vi "局部小信号变比.vi"(4 "长度":i32, 5 "数据":u8[](array[numeric]) format="%.0x") -> (3 "小信号变比":cluster{"UB":sgl, "IB":sgl, "UC":sgl, "IA":sgl})   [LabVIEW 2014]
panel:
  out "数组":u8[](array[numeric]) format="%x"
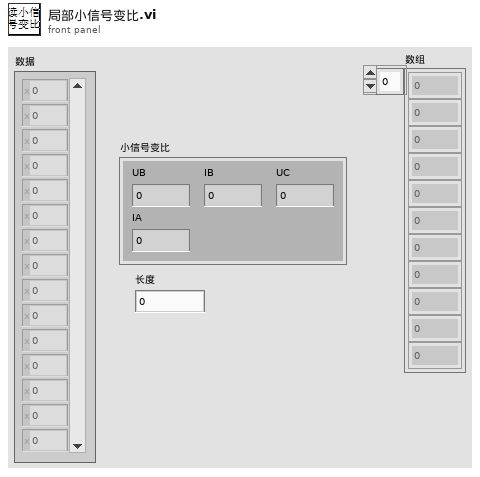
[diagram p1: front panel]
types:
  T1 = cluster{"有功常数":i32, "无功常数":i32, "输出类型":i32, "输出类型 2":i32}
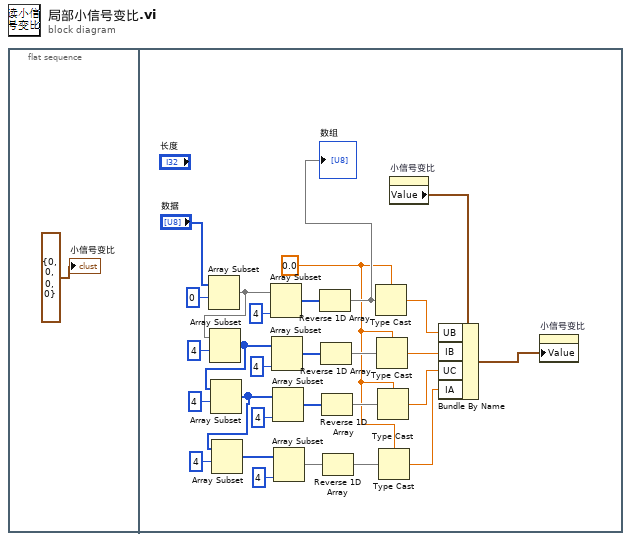
[diagram p0: block diagram]
diagram:
  n1 = flat-sequence {
    frame #0 {
      "小信号变比" <- T1 {"有功常数"=0, "无功常数"=0, "输出类型"=0, "输出类型 2"=0} ("本机表参数")
    }
    frame #1 {
      w3 = sgl 0.0
      n2 = Array Subset(array="数据", index=0 ("索引")) -> (w20:u8[])  [unwired: 1 in]
      n3 = Array Subset(array=w20, index=4 ("索引")) -> (w19:u8[])  [unwired: 1 in]
      n4 = Array Subset(array=w19, index=4 ("索引")) -> (w4:u8[])  [unwired: 1 in]
      n5 = Array Subset(array=w4, index=4 ("索引")) -> (w7:u8[])  [unwired: 1 in]
      n6 = Array Subset(array=w20, length=4 ("长度")) -> (w13:u8[])  [unwired: 1 in]
      n7 = Array Subset(array=w19, length=4 ("长度")) -> (w12:u8[])  [unwired: 1 in]
      n8 = Array Subset(array=w4, length=4 ("长度")) -> (w11:u8[])  [unwired: 1 in]
      n9 = Array Subset(array=w7, length=4 ("长度")) -> (w9:u8[])  [unwired: 1 in]
      n10 = Reverse 1D Array(array=w13) -> (reversed array=w10:u8[])
      "数组" <- w10
      n11 = Reverse 1D Array(array=w12) -> (reversed array=w26:u8[])
      n12 = Reverse 1D Array(array=w11) -> (reversed array=w21:u8[])
      n13 = Reverse 1D Array(array=w9) -> (reversed array=w8:u8[])
      n14 = Type Cast(type=w3, x=w10) -> (*(type *) &x=w15:sgl)
      n15 = Type Cast(type=w3, x=w26) -> (*(type *) &x=w18:sgl)
      n16 = Type Cast(type=w3, x=w21) -> (*(type *) &x=w16:sgl)
      n17 = Type Cast(type=w3, x=w8) -> (*(type *) &x=w2:sgl)
      n18 = property on="小信号变比" class="Clust (严格)"() -> ("Value"=w17:cluster{"UB":sgl, "IB":sgl, "UC":sgl, "IA":sgl})  [unwired: 2 in, 2 out]
      n19 = Bundle By Name(cluster=w17, "UB"=w15, "IB"=w18, "UC"=w16, "IA"=w2) -> (w14:cluster{"UB":sgl, "IB":sgl, "UC":sgl, "IA":sgl})
      n20 = property on="小信号变比" class="Clust (严格)"("Value"=w14) -> ()  [unwired: 2 in, 2 out]
    }
  }
